vi "Adc Conversion.vi"(8 "Error In":errorcluster, 10 "Numeric":dbl, 11 "Adc Convertor In":refnum<class "Adc Convertor.lvclass">) -> (0 "Error Out":errorcluster, 2 "Channel Data":T1, 3 "Adc Convertor Out":refnum<class "Adc Convertor.lvclass">)   [LabVIEW 2021, in "Adc Convertor.lvclass"]
doc: "This VI is an overriding method which performs the analog to digital conversion."
uses:
  Adc Convertor.lvclass
  Controls/Channel Data.ctl
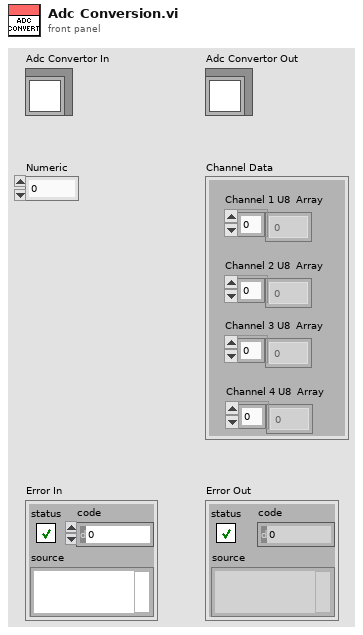
[diagram p1: front panel]
types:
  T1 = typedef "Channel Data.ctl" = cluster{"Channel 1 U8  Array":u8[], "Channel 2 U8  Array ":u8[], "Channel 3 U8  Array":u8[], "Channel 4 U8  Array":u8[]}
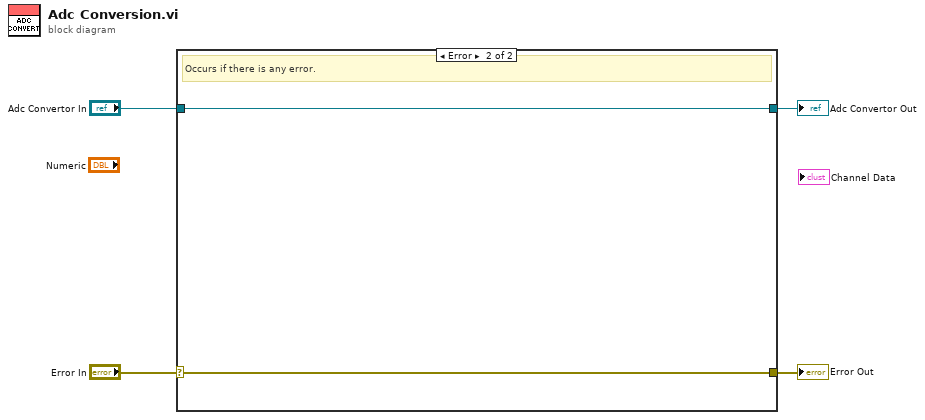
[diagram p0: block diagram]
diagram:
  n1 = case shown="Error" "Error In" {
    selector: "Error In" -> [w5 w8]
    tunnel: [w5 w8] -> w3
    tunnel: [w6 w7] -> w1
    tunnel: "Adc Convertor In" -> [w6 w7]
    frame No Error {
      # "Occurs if there is no error."
    }
    frame Error {
      # "Occurs if there is any error."
    }
  }
  "Error Out" <- w3
  "Adc Convertor Out" <- w1
